vi "Fractional-Year.vi"() -> (8 "Fractional Year":dbl format="%.3g")   [LabVIEW 2011]
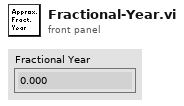
[diagram p1: front panel]
types:
  T1 = typedef "LVDateTimeRec.ctl" = cluster{"fractional second":dbl, "second":i32, "minute":i32, "hour":i32, "day of month":i32, "month":i32, "year":i32, "day of week":i32, "day of year":i32, "DST":i32}
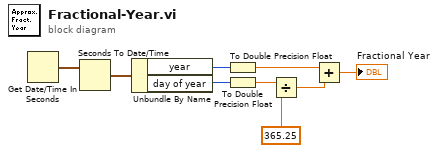
[diagram p0: block diagram]
diagram:
  n1 = Get Date/Time In Seconds() -> (seconds since 1Jan1904=w9:timestamp)
  n2 = Seconds To Date/Time(time stamp (now)=w9) -> (date time rec=w8:T1)  [unwired: 1 in]
  n3 = Unbundle By Name(w8) -> ("year"=w7:i32, "day of year"=w6:i32)
  n4 = To Double Precision Float(number=w7) -> (double precision float=w5:dbl)
  n5 = To Double Precision Float(number=w6) -> (double precision float=w1:dbl)
  n6 = Divide(x=w1, y=365.25) -> (x/y=w3:dbl)
  n7 = Add(x=w5, y=w3) -> (x+y=→"Fractional Year":dbl)
